vi "Convert spreadsheet string.vi"(6 "Delimiter [output]":string=",", 7 "Delimiter [input]":string=",", 8 "Format [output]":string="%^#_10e", 10 "List of numbers [input]":string="3479000000,3479100000,3479200000,3479300000,3479400000,3479500000,3479600000,3479700000,3479800000,3479900000,3480000000,3480100000,3480200000,3480300000,3480400000,3480500000,3480600000,3480700000,3480800000,3480900000,3481000000,3481100000,3481200000,3481300000,3481400000,3481500000,3481600000,3481700000,3481800000,3481900000,3482000000") -> (1 "Array [Dbl]":dbl[](array[numeric])=[3479000000.0, 3479100000.0, 3479200000.0, 3479300000.0, 3479400000.0, 3479500000.0, 3479600000.0, 3479700000.0, 3479800000.0, 3479900000.0, 3480000000.0, 3480100000.0, 3480200000.0, 3480300000.0, 3480400000.0, 3480500000.0, 3480600000.0, 3480700000.0, 3480800000.0, 3480900000.0, 3481000000.0, 3481100000.0, 3481200000.0, 3481300000.0, 3481400000.0, 3481500000.0, 3481600000.0, 3481700000.0, 3481800000.0, 3481900000.0, 3482000000.0], 2 "List of numbers [output]":string="3.479E+9,3.4791E+9,3.4792E+9,3.4793E+9,3.4794E+9,3.4795E+9,3.4796E+9,3.4797E+9,3.4798E+9,3.4799E+9,3.48E+9,3.4801E+9,3.4802E+9,3.4803E+9,3.4804E+9,3.4805E+9,3.4806E+9,3.4807E+9,3.4808E+9,3.4809E+9,3.481E+9,3.4811E+9,3.4812E+9,3.4813E+9,3.4814E+9,3.4815E+9,3.4816E+9,3.4817E+9,3.4818E+9,3.4819E+9,3.482E+9\r\n")   [LabVIEW 2019]
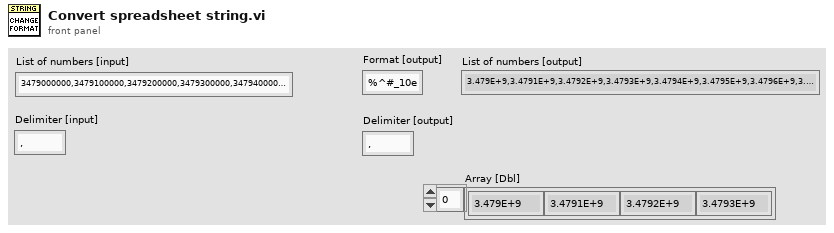
[diagram p1: front panel]
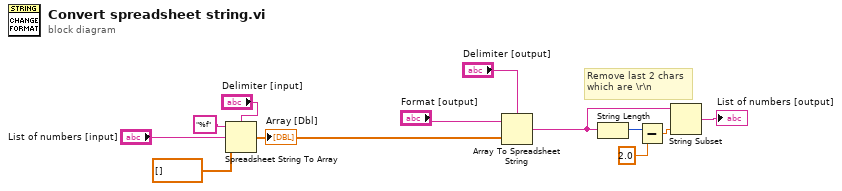
[diagram p0: block diagram]
diagram:
  # "Remove last 2 chars\nwhich are \\r\\n"
  n1 = Spreadsheet String To Array(delimiter (Tab)="Delimiter [input]", format string="%f", spreadsheet string="List of numbers [input]", array type (2D Dbl)=dbl[] []) -> (array=w8:dbl[])
  "Array [Dbl]" <- w8
  n2 = Array To Spreadsheet String(delimiter (Tab)="Delimiter [output]", array=w8, 3:"Format [output]") -> (spreadsheet string=w2:string)
  n3 = String Length(string=w2) -> (length=w3:i32)
  n4 = Subtract(x=w3, y=2.0) -> (x-y=w5:dbl)
  n5 = String Subset(string=w2, length (rest)=w5) -> (substring=→"List of numbers [output]":string)  [unwired: 1 in]
